vi "Get Project Ref.vi"(11 "CD Build Tools in":refnum<class "Project Sync Tools.lvclass">) -> (2 "Project Ref":refnum<vi>, 3 "CD Build Tools out":refnum<class "Project Sync Tools.lvclass">)   [LabVIEW 2019, in "Project Sync Tools.lvclass"]
uses:
  Project Sync Tools.lvclass
  Project Sync Tools.lvclass/Project Sync Tools.ctl
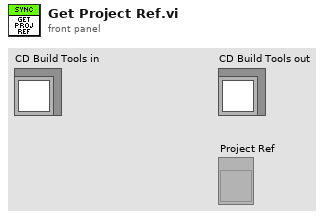
[diagram p1: front panel]
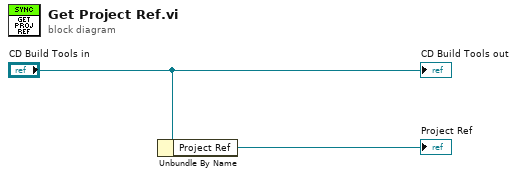
[diagram p0: block diagram]
diagram:
  n1 = Unbundle By Name("CD Build Tools in") -> ("Project Ref"=→"Project Ref":refnum<vi>)
  "CD Build Tools out" <- "CD Build Tools in"
